vi "Parameters UI - Dialog Box.vi"(0 "Parameters":string[][](array[string])) -> ()   [LabVIEW 2013]
uses:
  <vilib>/Utility/miscctls.llb/LVPointTypeDef.ctl
panel:
  in  "OK Button":bool
  out "Multicolumn Listbox":i32(listbox)=-1
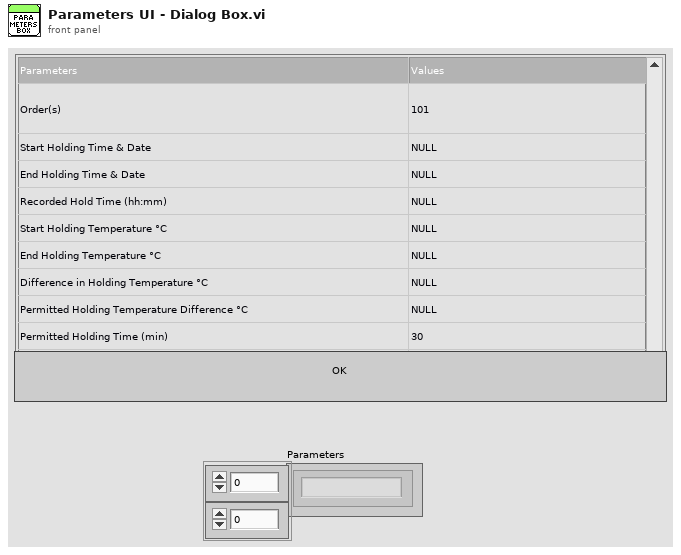
[diagram p1: front panel]
types:
  T1 = typedef "LVPointTypeDef.ctl" = cluster{"Horizontal":i16, "Vertical":i16}
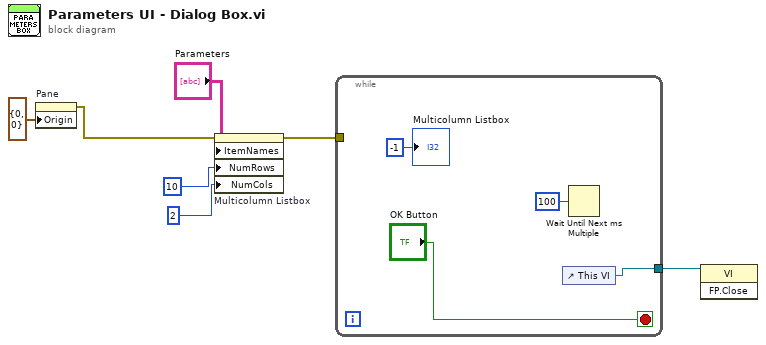
[diagram p0: block diagram]
diagram:
  n1 = property on="Pane" class="Pane"("Origin"=T1 {"Horizontal"=0, "Vertical"=0}) -> (error out=w1:errorcluster)  [unwired: 2 in, 1 out]
  n2 = property on="Multicolumn Listbox" class="MCListbox (strict)"(error in=w1, "ItemNames"="Parameters", "NumRows"=u32 10 ("Number of Rows"), "NumCols"=u32 2 ("Number of Columns")) -> (error out=w6:errorcluster)  [unwired: 1 in, 1 out]
  n3 = while {
    tunnel: [w9] -> w7
    tunnel: w6 -> [_]
    stop <- "OK Button" stop-if-true
    n4 = control-ref of="This VI"() -> (w9:refnum<vi>)
    n5 = Wait Until Next ms Multiple(millisecond multiple=u32 100) -> ()  [unwired: 1 out]
    "Multicolumn Listbox" <- -1 ("Multicolumn Listbox")
  }
  n6 = invoke class="VI" method="FP.Close"(reference=w7) -> ()  [unwired: 2 in, 3 out]
